vi "WriteConfigP.vi"(8 "error in (no error)":errorcluster) -> (0 "error out":errorcluster, 3 "Array":string[][](array[string]))   [LabVIEW 2020, in "Productos.lvlib"]
uses:
  Productos.lvlib
  <vilib>/Utility/xml.llb/Read From XML File(string).vi
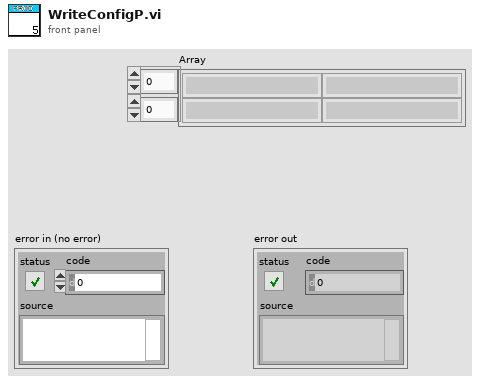
[diagram p1: front panel]
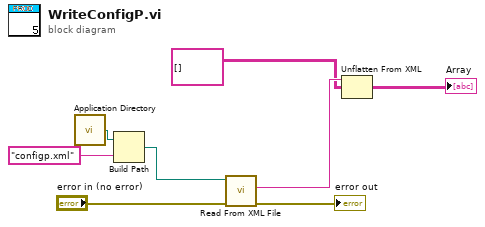
[diagram p0: block diagram]
diagram:
  n1 = call <vilib>:"Application Directory.vi"() -> ("Application Directory"=w7:path)
  n2 = Build Path(base path=w7, name or relative path="configp.xml") -> (appended path=w5:path)
  n3 = call-poly <vilib>:"Read From XML File.vi"("error in (no error)"="error in (no error)", "XML File Path"=w5) -> ("error out"=→"error out":errorcluster, "XML Elements"=w4:string)  [unwired: 7 in, 1 out]
  n4 = Unflatten From XML(xml string=w4, type=string[][] [] ("Array")) -> (value=→"Array":string[][])  [unwired: 1 in, 1 out]
